vi "From JSON.vi"(8 "error in":errorcluster, 10 "JSON":string, 11 "Theme Config in":refnum<class "Theme Config.lvclass">) -> (0 "error out":errorcluster, 3 "Theme Config out":refnum<class "Theme Config.lvclass">)   [LabVIEW 2021, in "Theme Config.lvclass"]
doc: "convert the class data into a json cluster for proper conversion\n\n<b>Code Developed By:</b>\nDaniel Coons\nTechnology Service Corporation\nwww.tsc.com/atcs"
uses:
  Theme Config.lvclass
  Theme Config.lvclass/Theme Config.ctl
  3422ac93-97d9-4446-a9c1-65bda130821d.vi
  <vilib>/JDP Science/JSONtext/JSON text to Variant.vi
  <vilib>/JDP Science/JSONtext/LVClass Serializer/JSONtext LVClass Serializer.lvclass
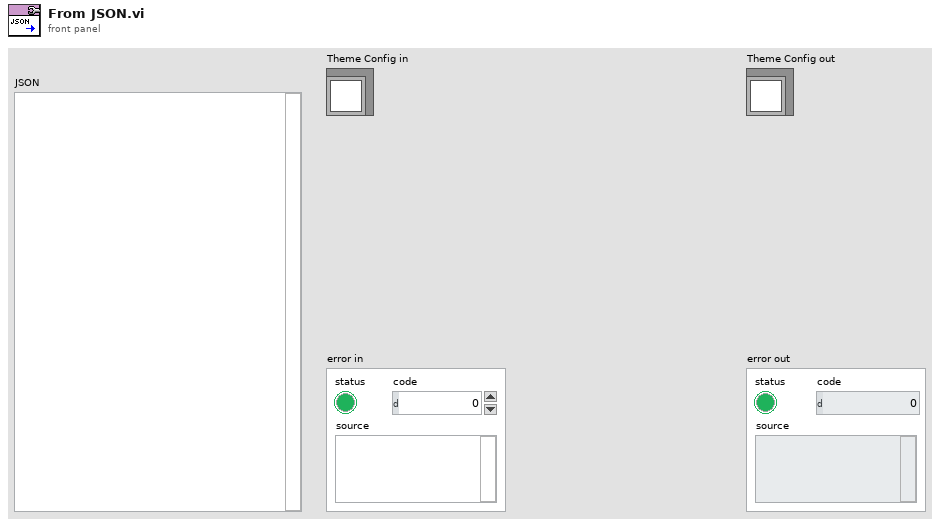
[diagram p1: front panel]
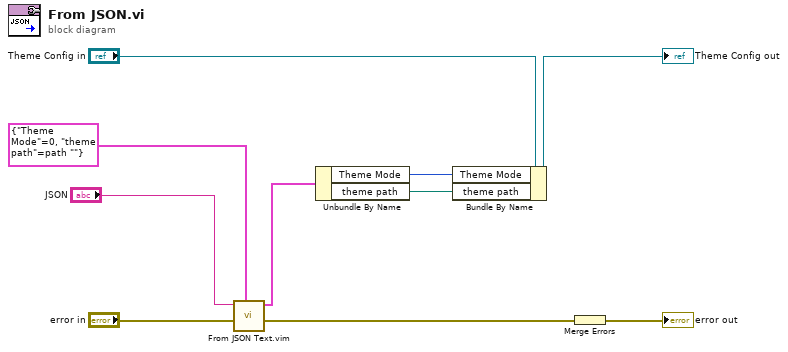
[diagram p0: block diagram]
diagram:
  n1 = call "From JSON Text.vim"("Data Type and Default Value"=cluster{"Theme Mode":u16, "theme path":path} {"Theme Mode"=0, "theme path"=path ""} ("Cluster of class private data"), "error in (no error)"="error in", "JSON"="JSON") -> ("error out"=w8:errorcluster, "Data out"=w3:cluster{"Theme Mode":u16, "theme path":path})  [unwired: 7 in]
  n2 = Unbundle By Name(w3) -> ("Theme Mode"=w2:u16, "theme path"=w1:path)
  n3 = Bundle By Name(cluster="Theme Config in", "Theme Mode"=w2, "theme path"=w1) -> (→"Theme Config out":refnum<class "Theme Config.lvclass">)
  n4 = Merge Errors(w8) -> (→"error out":errorcluster)
